vi "Write Power Meter.lvclass.vi"(10 "Power Meter classes":refnum<class "Power Meter.lvclass">[](array[class]), 11 "Harmonics in":refnum<class "Harmonics.lvclass">) -> (3 "Harmonics out":refnum<class "Harmonics.lvclass">)   [LabVIEW 2020, in "Harmonics.lvclass"]
uses:
  Harmonics.lvclass
  Instruments/Power Meter/Power Meter.lvclass
  Harmonics.lvclass/Harmonics.ctl
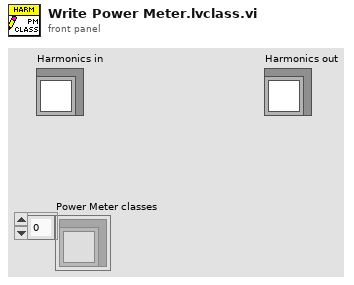
[diagram p1: front panel]
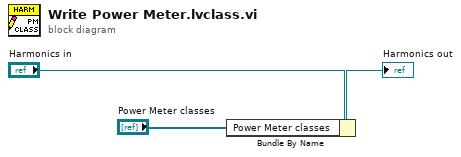
[diagram p0: block diagram]
diagram:
  n1 = Bundle By Name(cluster="Harmonics in", "Power Meter classes"="Power Meter classes") -> (→"Harmonics out":refnum<class "Harmonics.lvclass">)
